vi "Info From Config Data.vi"(7 "config data in":T2, 8 "error in (no error)":errorcluster, 9 "key":string, 10 "section":string, 11 "config data":T1) -> (0 "error out":errorcluster, 1 "key exists?":bool, 2 "section exists?":bool, 3 "config data out":T1, 4 "key index":i32, 5 "section index":i32, 6 "section contents":T3)   [LabVIEW 2009]
uses:
  Config Data Section.ctl
  Config Data.ctl
  <vilib>/Utility/config.llb/Config Data RefNum.ctl
  <vilib>/Utility/config.llb/NI_LVConfig.lvlib
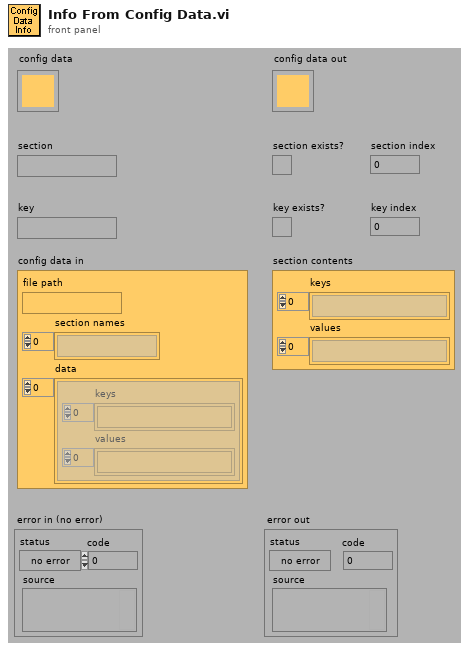
[diagram p1: front panel]
types:
  T1 = typedef "NI_LVConfig.lvlib/Config Data RefNum.ctl" = refnum<k1>
  T2 = typedef "Config Data.ctl" = cluster{"file path":path, "data":T3[], "section names":string[]}
  T3 = typedef "Config Data Section.ctl" = cluster{"keys":string[], "values":string[]}
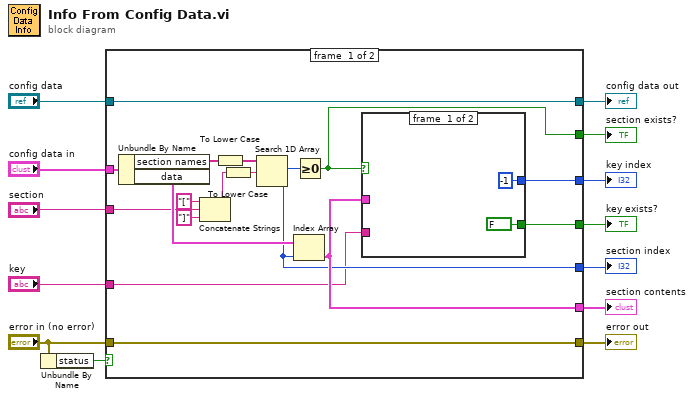
[diagram p0: block diagram]
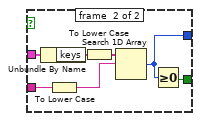
[diagram p2: hidden frame]
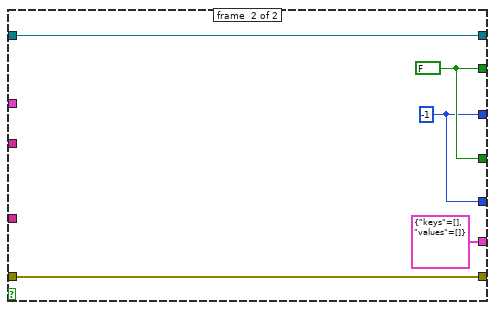
[diagram p3: hidden frame]
diagram:
  n1 = Unbundle By Name("error in (no error)") -> ("status"=w7:bool)
  n2 = case shown="False" w7 {
    tunnel: "config data in" -> [w30 _]
    tunnel: [w28 w43] -> w12
    tunnel: [w27 w42] -> w11
    tunnel: [w25 T3 {"keys"=[], "values"=[]} ("section")] -> w10
    tunnel: "section" -> [w21 _]
    tunnel: "error in (no error)" -> [w20 w41]
    tunnel: [w20 w41] -> w6
    tunnel: [w19 w44] -> w4
    tunnel: "config data" -> [w19 w44]
    tunnel: [w18 w43] -> w3
    tunnel: [w17 w42] -> w2
    tunnel: "key" -> [w16 _]
    frame #0 {
      n3 = Unbundle By Name(w30) -> ("section names"=w29:string[], "data"=w26:T3[])
      n4 = Concatenate Strings("[", w21, "]") -> (w22:string)
      n5 = To Lower Case(string=w29) -> (all lower case string=w15:string[])
      n6 = To Lower Case(string=w22) -> (all lower case string=w14:string)
      n7 = Search 1D Array(1D array=w15, element=w14) -> (index of element=w17:i32)  [unwired: 1 in]
      n8 = Index Array(array=w26, index=w17) -> (element=w25:T3)
      n9 = Greater Or Equal To 0?(x=w17) -> (x >= 0?=w18:bool)
      n10 = case shown="True" w18 {
        tunnel: [FALSE w36] -> w28
        tunnel: [-1 ("index of element") w35] -> w27
        tunnel: w25 -> [_ w39]
        tunnel: w16 -> [_ w37]
        frame #0 {
        }
        frame #1 {
          n11 = Unbundle By Name(w39) -> ("keys"=w38:string[])
          n12 = To Lower Case(string=w37) -> (all lower case string=w33:string)
          n13 = To Lower Case(string=w38) -> (all lower case string=w34:string[])
          n14 = Search 1D Array(1D array=w34, element=w33) -> (index of element=w35:i32)  [unwired: 1 in]
          n15 = Greater Or Equal To 0?(x=w35) -> (x >= 0?=w36:bool)
        }
      }
    }
    frame #1 {
      w42 = -1 ("index of element")
      w43 = FALSE
    }
  }
  "error out" <- w6
  "section exists?" <- w3
  "key exists?" <- w12
  "section index" <- w2
  "key index" <- w11
  "section contents" <- w10
  "config data out" <- w4
